vi "Get Port.vi"(8 "error in (no error)":errorcluster, 11 "Arduino in":refnum<class "Arduino.lvclass">) -> (0 "error out":errorcluster, 3 "Arduino out":refnum<class "Arduino.lvclass">)   [LabVIEW 2020, in "Arduino.lvclass"]
uses:
  Arduino.lvclass
  Abstract/Serial Device/Serial Device.lvclass
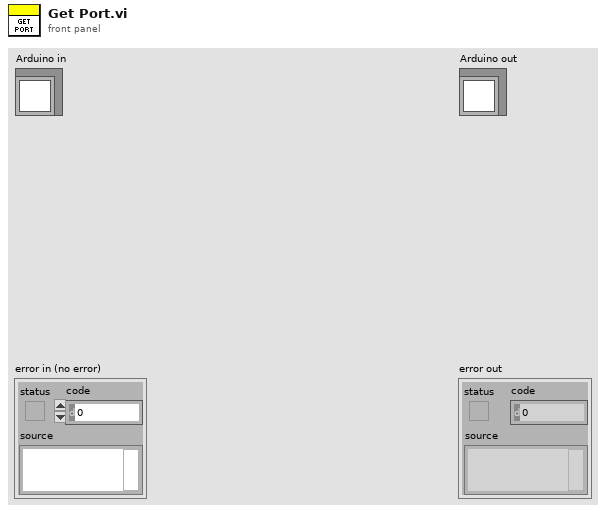
[diagram p1: front panel]
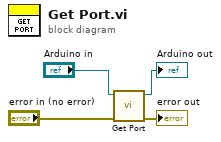
[diagram p0: block diagram]
diagram:
  n1 = call-parent "Get Port.vi"("error in (no error)"="error in (no error)", "Serial Device in"="Arduino in") -> ("error out"=→"error out":errorcluster, "Serial Device out"=→"Arduino out":refnum<class "Arduino.lvclass">)  [unwired: 8 in]
